vi "Delete.vi"(8 "error in (no error)":errorcluster, 11 "name":string) -> (0 "error out":errorcluster)   [LabVIEW 2017, in "DVRBuffer.lvlib"]
uses:
  <vilib>/addons/InsightCM/Devices/Shared/Common/DVRBuffer/DVRBuffer.lvlib
  <vilib>/addons/PointValueMap/PointValueMap.lvlib
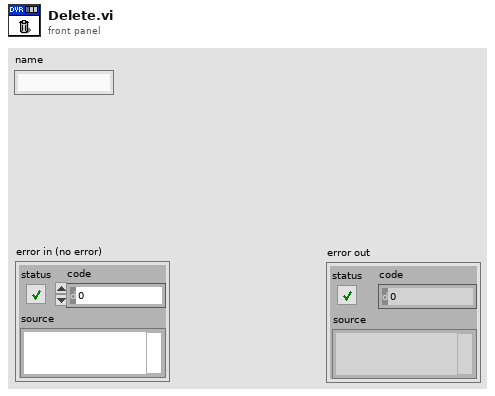
[diagram p1: front panel]
types:
  T1 = typedef "PointValueMap.lvlib/PointMap.ctl" = refnum<data-value>
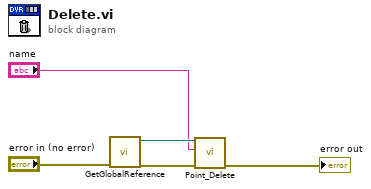
[diagram p0: block diagram]
diagram:
  n1 = call <vilib>:"GetGlobalReference.vi"("error in (no error)"="error in (no error)") -> ("error out"=w4:errorcluster, "reference"=w3:T1)  [unwired: 9 in]
  n2 = call <vilib>:"Point_Delete.vi"("Error In"=w4, "Tag"="name", "Map"=w3) -> ("Error Out"=→"error out":errorcluster)  [unwired: 7 in, 1 out]
